vi "Main.vi"() -> ()   [LabVIEW 2019]
doc: "The myRIO Project template acquires acceleration data from the onboard accelerometer and displays the changes of acceleration values in a waveform chart."
uses:
  <vilib>/myRIO/Instrument Drivers/Onboard Devices/Accelerometer/typedefs/Accelerometer Reference.ctl
  <vilib>/myRIO/Common/Instrument Driver Framework/Utilities/typedefs/myRIO Generic Hardware Reference.ctl
  <vilib>/myRIO/Common/Instrument Driver Framework/Utilities/typedefs/Hardware Version Enum.ctl
  <vilib>/myRIO/Common/Instrument Driver Framework/Utilities/typedefs/myRIO v1.0 Reference.ctl
  <vilib>/myRIO/Common/Instrument Driver Framework/Utilities/typedefs/Generic FPGA Reference.ctl
  <vilib>/myRIO/Common/Instrument Driver Framework/myRIO v1.0/Accelerometer/typedefs/Accelerometer Channels List.ctl
  <vilib>/myRIO/Common/Instrument Driver Framework/myRIO v1.0/Accelerometer/typedefs/Accelerometer Channels Enum.ctl
  <vilib>/userDefined/High Color/nirio_resource_hc.ctl
  <vilib>/myRIO/Instrument Drivers/Onboard IO/AO/typedefs/AO Reference.ctl
  <vilib>/myRIO/Common/Instrument Driver Framework/myRIO v1.0/AO/typedefs/AO Channels List.ctl
  <vilib>/myRIO/Common/Instrument Driver Framework/myRIO v1.0/AO/typedefs/AO Channels Enum.ctl
  <vilib>/myRIO/Common/Instrument Driver Framework/Utilities/typedefs/Analog Scaling Constants List.ctl
  <vilib>/myRIO/Common/Instrument Driver Framework/Utilities/typedefs/Analog Scaling Constants.ctl
  <vilib>/myRIO/Common/Instrument Driver Framework/Utilities/vis/Is FPGA Ref Available.vi
  <vilib>/myRIO/Common/Instrument Driver Framework/myRIO v1.0/Accelerometer/vis/myRIO v1.1 Open Accelerometer.vi
  <vilib>/myRIO/Instrument Drivers/Onboard Devices/Accelerometer/vis/Read.vi
  <vilib>/myRIO/Common/Instrument Driver Framework/myRIO v1.0/AO/vis/myRIO v1.1 Open AO.vi
  <vilib>/myRIO/Instrument Drivers/Onboard IO/AO/vis/Write.vi
  <vilib>/myRIO/Common/Instrument Driver Framework/Utilities/vis/Validate Channels.vi
  <vilib>/myRIO/Common/Instrument Driver Framework/myRIO v1.0/Accelerometer/vis/myRIO v1.0 Reserve Accelerometer.vi
  <vilib>/myRIO/Common/Instrument Driver Framework/myRIO v1.0/UART/vis/myRIO v1.0 Close UART.vi
  <vilib>/myRIO/Common/Instrument Driver Framework/myRIO v1.0/AO/vis/myRIO v1.0 Reserve AO.vi
  <vilib>/myRIO/Common/Instrument Driver Framework/myRIO v1.0/Resource Manager/vis/myRIO v1.0 Reserve Channel List.vi
  <vilib>/myRIO/Common/Instrument Driver Framework/myRIO v1.0/Accelerometer/vis/myRIO v1.0 Build MUX Configuration Accelerometer.vi
  <vilib>/myRIO/Common/Instrument Driver Framework/myRIO v1.0/AO/vis/myRIO v1.0 Build MUX Configuration AO.vi
  <vilib>/myRIO/Common/Instrument Driver Framework/myRIO v1.0/Resource Manager/vis/myRIO v1.0 Reserve Channel.vi
  <vilib>/myRIO/Common/Instrument Driver Framework/myRIO v1.0/Resource Manager/vis/myRIO v1.0 Unreserve Channel.vi
  <vilib>/myRIO/Common/Instrument Driver Framework/myRIO v1.0/Resource Manager/vis/myRIO v1.0 Build Mutex Name.vi
  <vilib>/Utility/VariantDataType/GetNumericInfo.vi
  <vilib>/Utility/error.llb/Error Cluster From Error Code.vi
  <vilib>/myRIO/Common/Instrument Driver Framework/myRIO v1.0/myRIO v1.1 Open.vi
  <vilib>/myRIO/Common/Instrument Driver Framework/myRIO v1.0/AO/vis/myRIO v1.0 Get Scaling Constants AO.vi
  <vilib>/myRIO/Common/Instrument Driver Framework/Utilities/vis/IO Manager.vi
  <vilib>/myRIO/Common/Instrument Driver Framework/Utilities/vis/Configuration Manager.vi
  <vilib>/myRIO/Common/Instrument Driver Framework/myRIO v1.0/myRIO v1.0 Close.vi
  <vilib>/myRIO/Common/Instrument Driver Framework/myRIO v1.0/AO/vis/myRIO v1.0 Write AO.vi
  <vilib>/myRIO/Common/Instrument Driver Framework/myRIO v1.0/Accelerometer/vis/myRIO v1.0 Get Scaling Constant Accelerometer.vi
  <vilib>/myRIO/Common/Instrument Driver Framework/myRIO v1.0/Accelerometer/vis/myRIO v1.0 Read Accelerometer.vi
  <vilib>/myRIO/Common/Instrument Driver Framework/Utilities/vis/FPGA Ref Manager.vi
  <vilib>/myRIO/Common/Instrument Driver Framework/myRIO v1.0/myRIO v1.0 Reset FPGA.vi
  <vilib>/myRIO/Common/Instrument Driver Framework/myRIO v1.0/IRQ/vis/myRIO v1.0 IRQ Info FGV.vi
  <vilib>/myRIO/Common/Instrument Driver Framework/myRIO v1.0/IRQ/vis/myRIO v1.0 Timer IRQ Info FGV.vi
  <vilib>/myRIO/Common/Instrument Driver Framework/myRIO v1.0/IRQ/vis/myRIO v1.0 ISR Agent.vi
  <vilib>/myRIO/Instrument Drivers/Utilities/vis/Reset Index.vi
  <vilib>/myRIO/Common/Instrument Driver Framework/myRIO v1.0/Resource Manager/vis/myRIO v1.0 Block Write Resource Manager.vi
  <vilib>/myRIO/Express VI/Onboard IO/AO/AO Express VI.xnode
  <vilib>/myRIO/Instrument Drivers/Onboard IO/AO/vis/myRIO AO Open.xnode
  <vilib>/myRIO/Express VI/Onboard Devices/Accelerometer/Accelerometer Express VI.xnode
  <vilib>/myRIO/Instrument Drivers/Onboard Devices/Accelerometer/vis/myRIO Accelerometer Open.xnode
  <vilib>/myRIO/Instrument Drivers/Utilities/Utilities.lvlib
  <vilib>/myRIO/Instrument Drivers/Onboard Devices/Accelerometer/Accelerometer.lvlib
  <vilib>/myRIO/Instrument Drivers/Onboard IO/AO/AO.lvlib
panel:
  in  "Numeric 4":dbl
  in  "Numeric 3":dbl
  out "Array":i32[](array[numeric])
  in  "input array   4":dbl[](array[numeric])
  out "Numeric":i32
  out "Acceleration":T1(graph)
  out "error out":errorcluster
  in  "Stop":bool
  # "Overview: The myRIO Project template acquires acceleration data from the onboard accelerometer and displays the changes of acceleration values in a waveform chart.\nInstructions:\n1. Check the myRIO target IP address in the project and make sure the target IP address is correct. \n2. Run this VI."
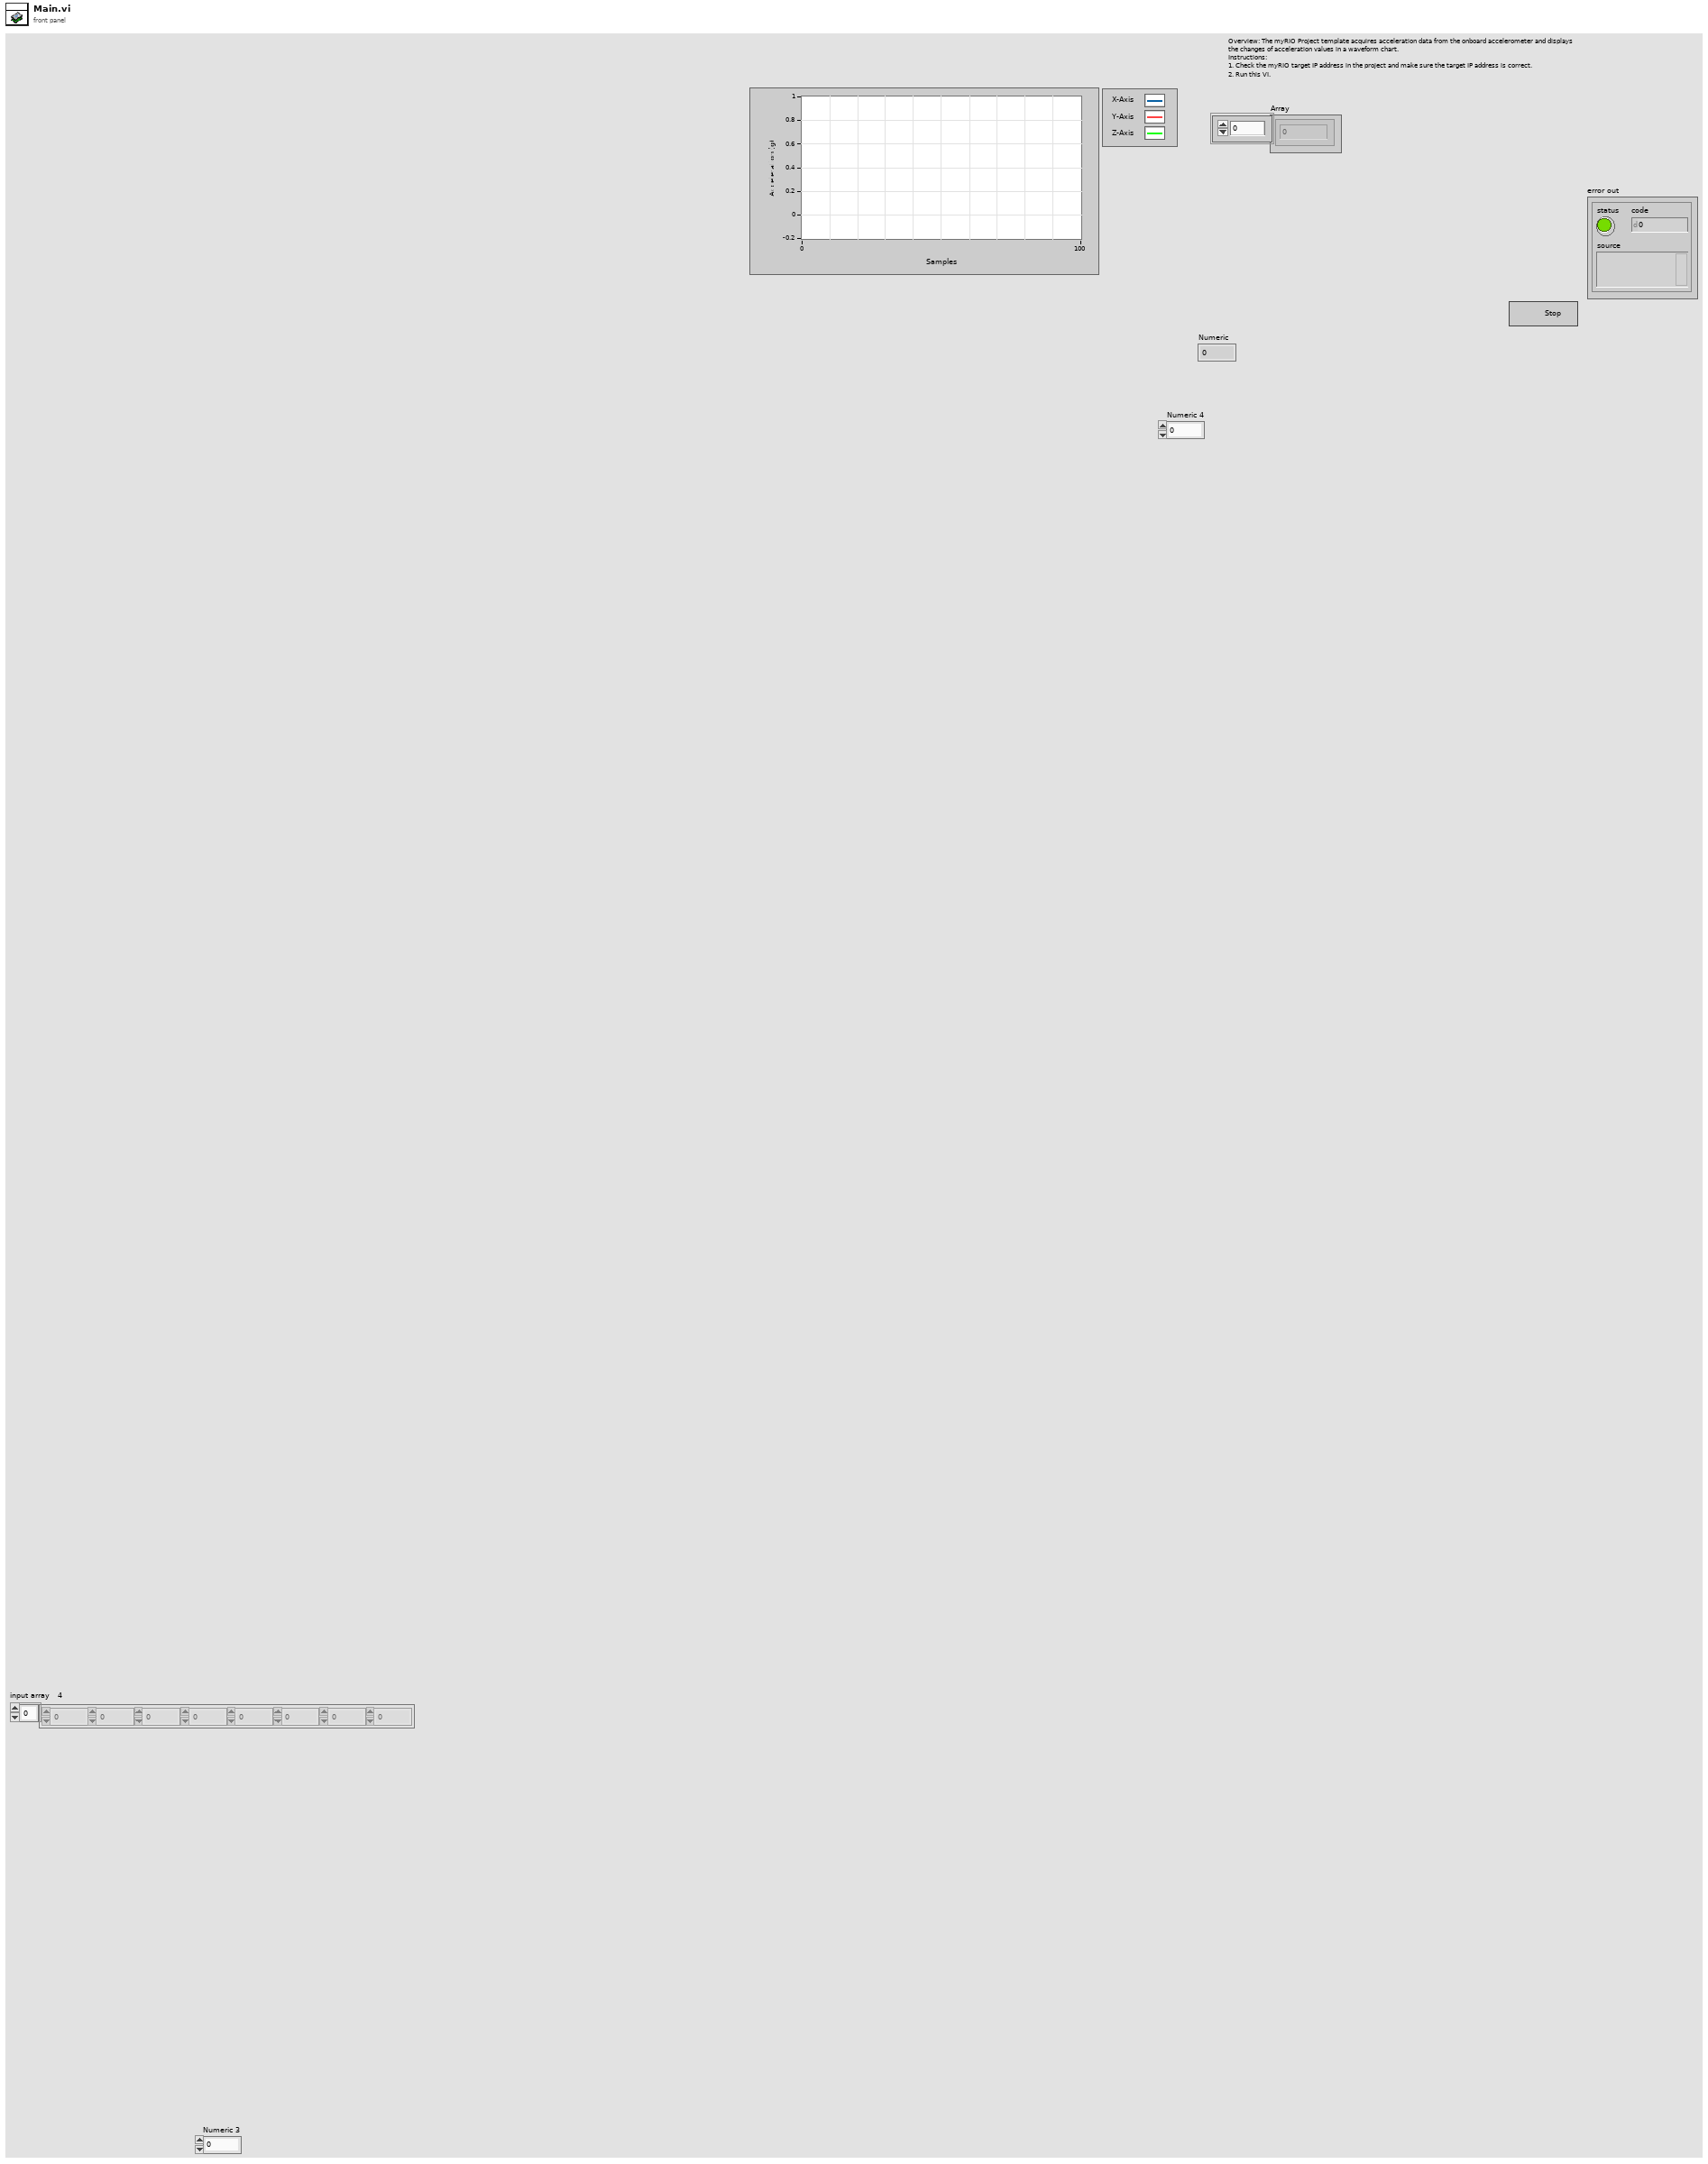
[diagram p1: front panel]
types:
  T1 = cluster{"X-Axis":dbl, "Y-Axis":dbl, "Z-Axis":dbl}
  T2 = typedef "Accelerometer.lvlib/Accelerometer Reference.ctl" = cluster{"myRIO Reference":T3, "Accelerometer Channels List":T7, "LSB Weight":dbl}
  T3 = typedef "myRIO Generic Hardware Reference.ctl" = cluster{"myRIO Model":T4, "myRIO Hardware Reference":T5}
  T4 = typedef "Hardware Version Enum.ctl" = enum16{"Unknown", "myRIO-1900", "myRIO-1950", "roboRIO", "NI ELVIS RIO CM", "ELVIS III"}
  T5 = typedef "myRIO v1.0 Reference.ctl" = cluster{"Generic FPGA Reference":T6, "Allow multiple opens":bool}
  T6 = typedef "Generic FPGA Reference.ctl" = refnum<k20>
  T7 = typedef "Accelerometer Channels List.ctl" = T8[]
  T8 = typedef "Accelerometer Channels Enum.ctl" = enum16{"Not Connected", "X-Axis", "Y-Axis", "Z-Axis"}
  T9 = typedef "nirio_resource_hc.ctl" = tag
  T10 = typedef "AO.lvlib/AO Reference.ctl" = cluster{"myRIO Reference":T3, "AO Channel List":T11, "AO Scaling Constant List":T13}
  T11 = typedef "AO Channels List.ctl" = T12[]
  T12 = typedef "AO Channels Enum.ctl" = enum16{"Not Connected", "AudioOut/Left", "AudioOut/Right", "C/AO0", "C/AO1", "A/AO0", "A/AO1", "B/AO0", "B/AO1"}
  T13 = typedef "Analog Scaling Constants List.ctl" = T14[]
  T14 = typedef "Analog Scaling Constants.ctl" = cluster{"LSB Weight (Volts)":dbl, "Offset (Volts)":dbl, "Signed?":bool}
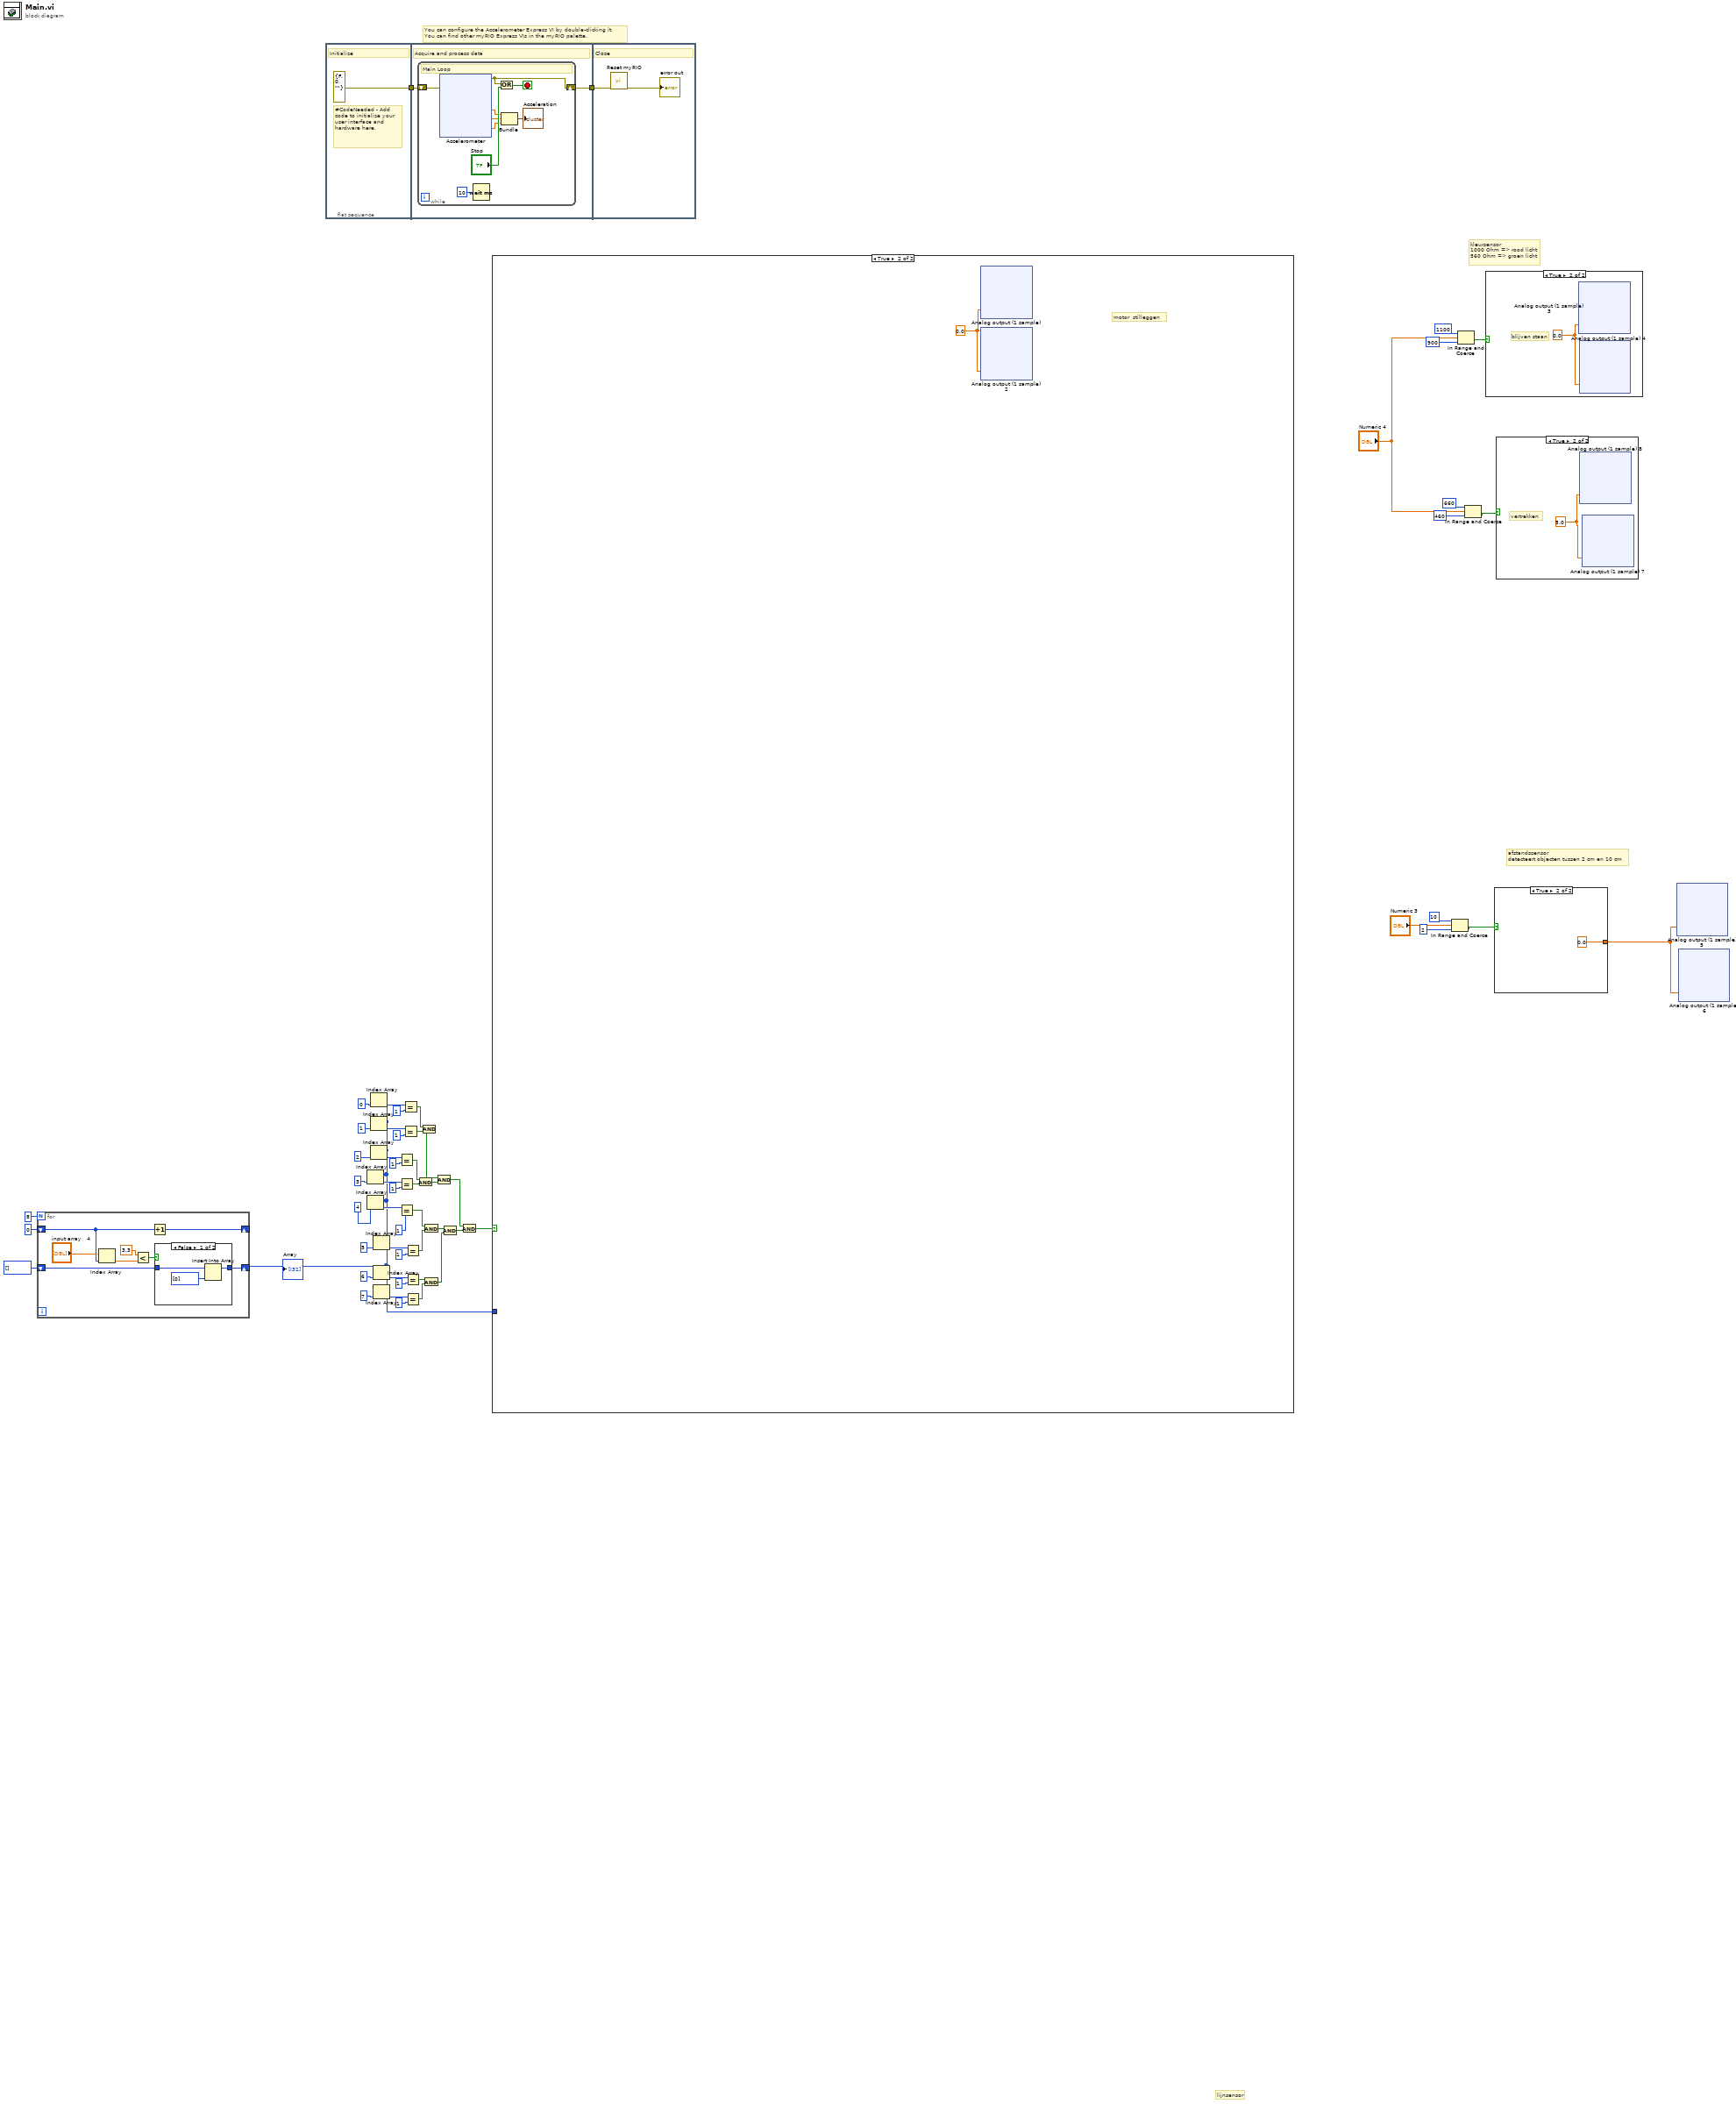
[diagram p0: block diagram]
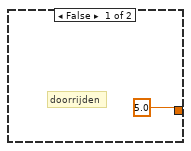
[diagram p4: hidden frame]
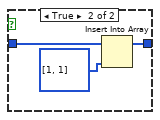
[diagram p5: hidden frame]
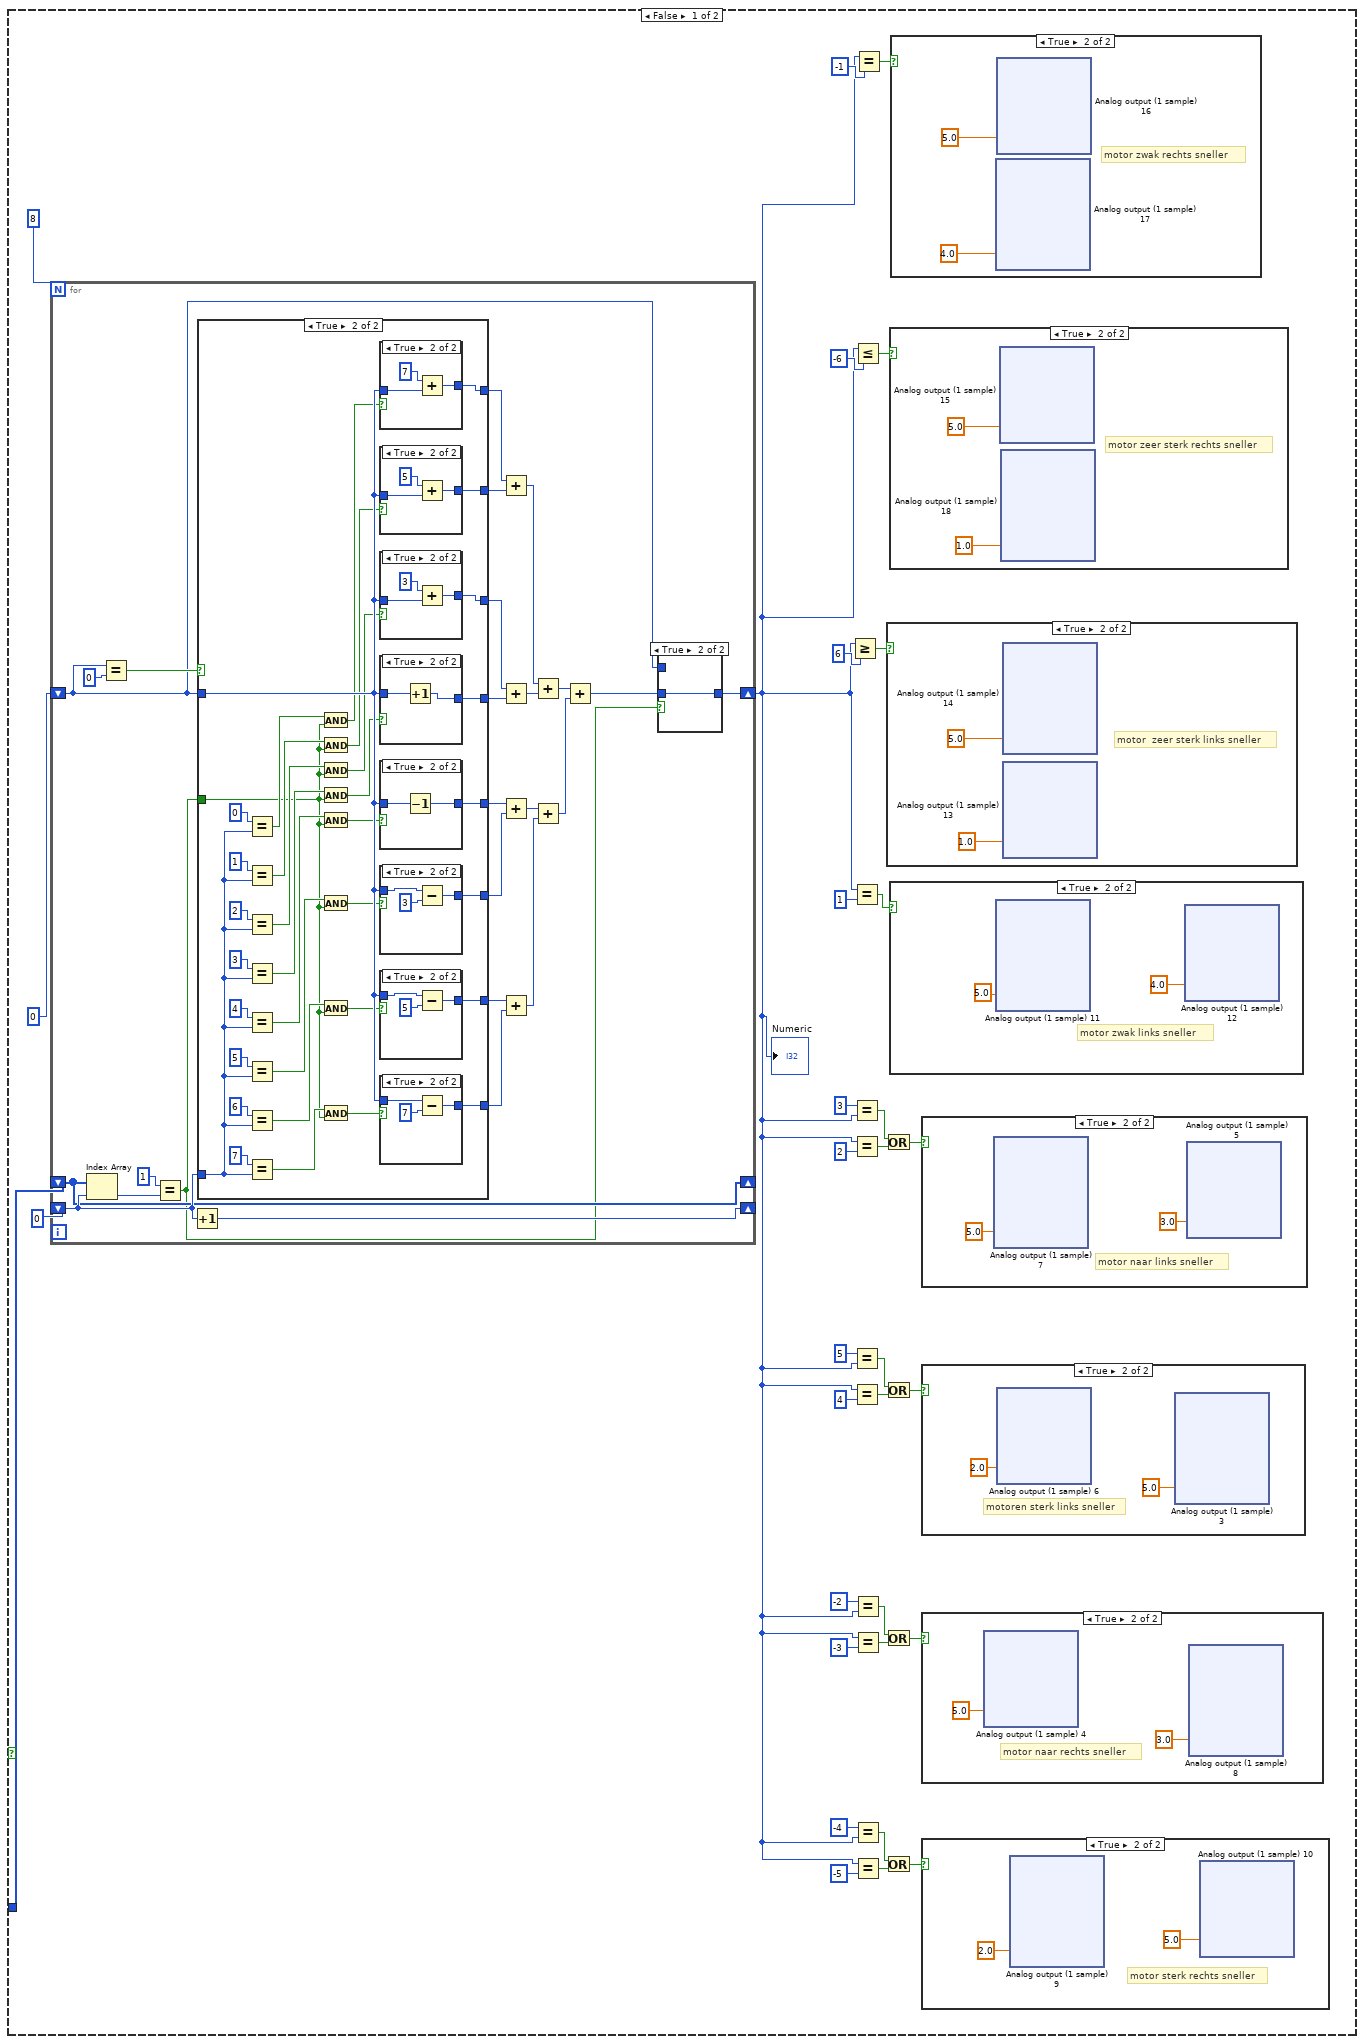
[diagram p6: hidden frame]
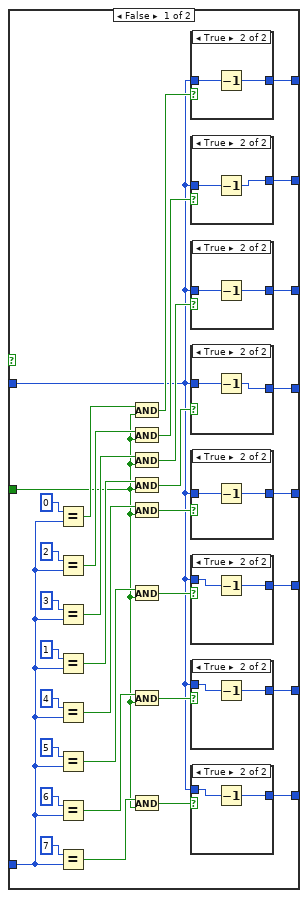
[diagram p16: hidden frame]
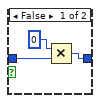
[diagram p17: hidden frame]
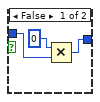
[diagram p18: hidden frame]
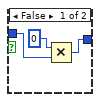
[diagram p19: hidden frame]
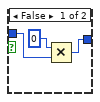
[diagram p20: hidden frame]
diagram:
  # "kleursensor    \n1000 Ohm => rood licht\n560 Ohm => groen licht"
  # "afstandssensor\ndetecteert objecten tussen 2 cm en 10 cm"
  # "lijnsensor"
  # "You can configure the Accelerometer Express VI by double-clicking it.\nYou can find other myRIO Express VIs in the myRIO palette."
  n1 = for {
    N: 8 -> [_]
    shift-right: [w64] -> w13
    shift-left: i32[] [] -> [w65]
    shift-right: [w61] -> _
    shift-left: 0 -> [w60]
    n2 = Index Array(array="input array   4", index=w60) -> (element=w58:dbl)
    n3 = Less?(x=3.3, y=w58) -> (x < y?=w63:bool)
    n4 = Increment(x=w60) -> (x+1=w61:i32)
    n5 = case shown="False" w63 {
      tunnel: w65 -> [w67 w69]
      tunnel: [w68 w71] -> w64
      frame False {
        n6 = Insert Into Array(array=w67, new element=i32[] [0]) -> (w68:i32[])  [unwired: 1 in]
      }
      frame True {
        n7 = Insert Into Array(array=w69, new element=i32[] [1, 1]) -> (w71:i32[])  [unwired: 1 in]
      }
    }
  }
  "Array" <- w13
  n8 = flat-sequence {
    tunnel: [errorcluster {"status"=FALSE, "code"=0, "source"=""} ("error in (no error)")] -> w57
    tunnel: w57 -> [w74]
    tunnel: [w73] -> w56
    tunnel: w56 -> [w124]
    frame #0 {
      # "#CodeNeeded - Add code to initialize your user interface and hardware here."
      # "Initialize"
    }
    frame #1 {
      # "Acquire and process data"
      n9 = while {
        shift-right: [w78] -> w73
        shift-left: w74 -> [w79]
        stop <- w82 stop-if-true
        # "Main Loop"
        n10 = xnode "Accelerometer"("error in (no error)"=w79) -> ("X-Axis"=w77:dbl, "Y-Axis"=w76:dbl, "Z-Axis"=w75:dbl, "error out"=w78:errorcluster)
        n11 = Wait (ms)(milliseconds to wait=u32 10) -> ()  [unwired: 1 out]
        n12 = Or(x=w78, y="Stop") -> (x .or. y?=w82:bool)
        n13 = Bundle("X-Axis"=w77, "Y-Axis"=w76, "Z-Axis"=w75) -> (→"Acceleration":T1)  [unwired: 1 in]
      }
    }
    frame #2 {
      # "Close"
      n14 = call <vilib>:"Reset myRIO.vi"("error in (no error)"=w124) -> ("error out"=→"error out":errorcluster)  [unwired: 10 in]
    }
  }
  n15 = Index Array(array=w13, index=3) -> (element=w52:i32)
  n16 = Index Array(array=w13, index=4) -> (element=w46:i32)
  n17 = Index Array(array=w13, index=0) -> (element=w34:i32)
  n18 = Index Array(array=w13, index=1) -> (element=w55:i32)
  n19 = Index Array(array=w13, index=2) -> (element=w49:i32)
  n20 = Index Array(array=w13, index=5) -> (element=w43:i32)
  n21 = Index Array(array=w13, index=6) -> (element=w40:i32)
  n22 = Index Array(array=w13, index=7) -> (element=w37:i32)
  n23 = Equal?(x=w49, y=1) -> (x = y?=w29:bool)
  n24 = Equal?(x=w52, y=1) -> (x = y?=w28:bool)
  n25 = Equal?(x=w46, y=1) -> (x = y?=w27:bool)
  n26 = Equal?(x=w34, y=1) -> (x = y?=w31:bool)
  n27 = Equal?(x=w55, y=1) -> (x = y?=w30:bool)
  n28 = Equal?(x=w43, y=1) -> (x = y?=w26:bool)
  n29 = Equal?(x=w40, y=1) -> (x = y?=w25:bool)
  n30 = Equal?(x=w37, y=1) -> (x = y?=w24:bool)
  n31 = And(x=w29, y=w28) -> (x .and. y?=w22:bool)
  n32 = And(x=w31, y=w30) -> (x .and. y?=w23:bool)
  n33 = And(x=w27, y=w26) -> (x .and. y?=w21:bool)
  n34 = And(x=w25, y=w24) -> (x .and. y?=w20:bool)
  n35 = And(x=w23, y=w22) -> (x .and. y?=w19:bool)
  n36 = And(x=w21, y=w20) -> (x .and. y?=w18:bool)
  n37 = And(x=w19, y=w18) -> (x .and. y?=w17:bool)
  n38 = case shown="True" w17 {
    tunnel: w13 -> [w126 _]
    frame False {
      n39 = for {
        N: 8 -> [_]
        shift-right: [w776] -> _
        shift-left: 0 -> [w790]
        shift-right: [w768] -> w125
        shift-left: 0 -> [w769]
        shift-right: [w781] -> _
        shift-left: w126 -> [w781]
        n40 = Index Array(array=w781, index=w790) -> (element=w780:i32)
        n41 = Equal?(x=w769, y=0) -> (x = y?=w777:bool)
        n42 = Equal?(x=1, y=w780) -> (x = y?=w767:bool)
        n43 = Increment(x=w790) -> (x+1=w776:i32)
        n44 = case shown="True" w777 {
          tunnel: w790 -> [w800 w886]
          tunnel: [w794 w885] -> w789
          tunnel: [w801 w884] -> w788
          tunnel: [w802 w883] -> w787
          tunnel: [w803 w882] -> w786
          tunnel: w769 -> [w793 w881]
          tunnel: w767 -> [w799 w872]
          tunnel: [w797 w871] -> w775
          tunnel: [w798 w870] -> w774
          tunnel: [w795 w869] -> w772
          tunnel: [w796 w868] -> w771
          frame False {
            n45 = Equal?(x=0, y=w800) -> (x = y?=w820:bool)
            n46 = Equal?(x=2, y=w800) -> (x = y?=w826:bool)
            n47 = Equal?(x=3, y=w800) -> (x = y?=w827:bool)
            n48 = Equal?(x=1, y=w800) -> (x = y?=w812:bool)
            n49 = Equal?(x=4, y=w800) -> (x = y?=w824:bool)
            n50 = Equal?(x=5, y=w800) -> (x = y?=w825:bool)
            n51 = Equal?(x=6, y=w800) -> (x = y?=w823:bool)
            n52 = Equal?(x=7, y=w800) -> (x = y?=w822:bool)
            n53 = And(x=w820, y=w799) -> (x .and. y?=w804:bool)
            n54 = And(x=w826, y=w799) -> (x .and. y?=w806:bool)
            n55 = And(x=w827, y=w799) -> (x .and. y?=w807:bool)
            n56 = And(x=w812, y=w799) -> (x .and. y?=w805:bool)
            n57 = And(x=w824, y=w799) -> (x .and. y?=w808:bool)
            n58 = And(x=w825, y=w799) -> (x .and. y?=w809:bool)
            n59 = And(x=w823, y=w799) -> (x .and. y?=w810:bool)
            n60 = And(x=w822, y=w799) -> (x .and. y?=w811:bool)
            n61 = case shown="True" w804 {
              tunnel: [w829 w832] -> w798
              tunnel: w793 -> [w828 w831]
              frame False {
                n62 = Multiply(x=0, y=w828) -> (x*y=w829:i32)
              }
              frame True {
                n63 = Decrement(x=w831) -> (x-1=w832:i32)
              }
            }
            n64 = case shown="True" w806 {
              tunnel: [w860 w861] -> w797
              tunnel: w793 -> [w859 w862]
              frame False {
                n65 = Multiply(x=0, y=w859) -> (x*y=w860:i32)
              }
              frame True {
                n66 = Decrement(x=w862) -> (x-1=w861:i32)
              }
            }
            n67 = case shown="True" w807 {
              tunnel: [w854 w857] -> w796
              tunnel: w793 -> [w853 w856]
              frame False {
                n68 = Multiply(x=0, y=w853) -> (x*y=w854:i32)
              }
              frame True {
                n69 = Decrement(x=w856) -> (x-1=w857:i32)
              }
            }
            n70 = case shown="True" w805 {
              tunnel: [w864 w867] -> w795
              tunnel: w793 -> [w863 w866]
              frame False {
                n71 = Multiply(x=0, y=w863) -> (x*y=w864:i32)
              }
              frame True {
                n72 = Decrement(x=w866) -> (x-1=w867:i32)
              }
            }
            n73 = case shown="True" w808 {
              tunnel: [w849 w852] -> w794
              tunnel: w793 -> [w848 w851]
              frame False {
                n74 = Multiply(x=0, y=w848) -> (x*y=w849:i32)
              }
              frame True {
                n75 = Decrement(x=w851) -> (x-1=w852:i32)
              }
            }
            n76 = case shown="True" w809 {
              tunnel: [w839 w842] -> w801
              tunnel: w793 -> [w838 w841]
              frame False {
                n77 = Multiply(x=0, y=w838) -> (x*y=w839:i32)
              }
              frame True {
                n78 = Decrement(x=w841) -> (x-1=w842:i32)
              }
            }
            n79 = case shown="True" w810 {
              tunnel: [w844 w847] -> w802
              tunnel: w793 -> [w843 w846]
              frame False {
                n80 = Multiply(x=0, y=w843) -> (x*y=w844:i32)
              }
              frame True {
                n81 = Decrement(x=w846) -> (x-1=w847:i32)
              }
            }
            n82 = case shown="True" w811 {
              tunnel: [w833 w837] -> w803
              tunnel: w793 -> [w834 w836]
              frame False {
                n83 = Multiply(x=0, y=w834) -> (x*y=w833:i32)
              }
              frame True {
                n84 = Decrement(x=w836) -> (x-1=w837:i32)
              }
            }
          }
          frame True {
            n85 = Equal?(x=0, y=w886) -> (x = y?=w895:bool)
            n86 = Equal?(x=1, y=w886) -> (x = y?=w887:bool)
            n87 = Equal?(x=2, y=w886) -> (x = y?=w901:bool)
            n88 = Equal?(x=3, y=w886) -> (x = y?=w902:bool)
            n89 = Equal?(x=4, y=w886) -> (x = y?=w899:bool)
            n90 = Equal?(x=5, y=w886) -> (x = y?=w900:bool)
            n91 = Equal?(x=6, y=w886) -> (x = y?=w898:bool)
            n92 = Equal?(x=7, y=w886) -> (x = y?=w897:bool)
            n93 = And(x=w895, y=w872) -> (x .and. y?=w873:bool)
            n94 = And(x=w887, y=w872) -> (x .and. y?=w874:bool)
            n95 = And(x=w901, y=w872) -> (x .and. y?=w875:bool)
            n96 = And(x=w902, y=w872) -> (x .and. y?=w876:bool)
            n97 = And(x=w899, y=w872) -> (x .and. y?=w877:bool)
            n98 = And(x=w900, y=w872) -> (x .and. y?=w878:bool)
            n99 = And(x=w898, y=w872) -> (x .and. y?=w879:bool)
            n100 = And(x=w897, y=w872) -> (x .and. y?=w880:bool)
            n101 = case shown="True" w873 {
              tunnel: w881 -> [w903 w907]
              tunnel: [w904 w906] -> w870
              frame False {
                n102 = Multiply(x=0, y=w903) -> (x*y=w904:i32)
              }
              frame True {
                n103 = Add(x=7, y=w907) -> (x+y=w906:i32)
              }
            }
            n104 = case shown="True" w874 {
              tunnel: w881 -> [w943 w946]
              tunnel: [w944 w947] -> w871
              frame False {
                n105 = Multiply(x=0, y=w943) -> (x*y=w944:i32)
              }
              frame True {
                n106 = Add(x=5, y=w946) -> (x+y=w947:i32)
              }
            }
            n107 = case shown="True" w875 {
              tunnel: w881 -> [w937 w941]
              tunnel: [w938 w940] -> w868
              frame False {
                n108 = Multiply(x=0, y=w937) -> (x*y=w938:i32)
              }
              frame True {
                n109 = Add(x=3, y=w941) -> (x+y=w940:i32)
              }
            }
            n110 = case shown="True" w876 {
              tunnel: w881 -> [w933 w936]
              tunnel: [w932 w935] -> w869
              frame False {
                n111 = Multiply(x=0, y=w933) -> (x*y=w932:i32)
              }
              frame True {
                n112 = Increment(x=w936) -> (x+1=w935:i32)
              }
            }
            n113 = case shown="True" w877 {
              tunnel: w881 -> [w927 w931]
              tunnel: [w928 w930] -> w885
              frame False {
                n114 = Multiply(x=0, y=w927) -> (x*y=w928:i32)
              }
              frame True {
                n115 = Decrement(x=w931) -> (x-1=w930:i32)
              }
            }
            n116 = case shown="True" w878 {
              tunnel: w881 -> [w916 w918]
              tunnel: [w915 w920] -> w884
              frame False {
                n117 = Multiply(x=0, y=w916) -> (x*y=w915:i32)
              }
              frame True {
                n118 = Subtract(x=w918, y=3) -> (x-y=w920:i32)
              }
            }
            n119 = case shown="True" w879 {
              tunnel: w881 -> [w922 w924]
              tunnel: [w921 w925] -> w883
              frame False {
                n120 = Multiply(x=0, y=w922) -> (x*y=w921:i32)
              }
              frame True {
                n121 = Subtract(x=w924, y=5) -> (x-y=w925:i32)
              }
            }
            n122 = case shown="True" w880 {
              tunnel: w881 -> [w909 w912]
              tunnel: [w910 w913] -> w882
              frame False {
                n123 = Multiply(x=0, y=w909) -> (x*y=w910:i32)
              }
              frame True {
                n124 = Subtract(x=w912, y=7) -> (x-y=w913:i32)
              }
            }
          }
        }
        n125 = Add(x=w774, y=w775) -> (x+y=w773:i32)
        n126 = Add(x=w771, y=w772) -> (x+y=w770:i32)
        n127 = Add(x=w789, y=w788) -> (x+y=w784:i32)
        n128 = Add(x=w787, y=w786) -> (x+y=w785:i32)
        n129 = Add(x=w773, y=w770) -> (x+y=w783:i32)
        n130 = Add(x=w784, y=w785) -> (x+y=w782:i32)
        n131 = Add(x=w783, y=w782) -> (x+y=w766:i32)
        n132 = case shown="True" w767 {
          tunnel: w769 -> [w791 _]
          tunnel: [w791 w792] -> w768
          tunnel: w766 -> [_ w792]
          frame False {
          }
          frame True {
          }
        }
      }
      "Numeric" <- w125
      n133 = Greater Or Equal?(x=w125, y=6) -> (x >= y?=w152:bool)
      n134 = Equal?(x=w125, y=1) -> (x = y?=w153:bool)
      n135 = Equal?(x=3, y=w125) -> (x = y?=w143:bool)
      n136 = Equal?(x=w125, y=2) -> (x = y?=w144:bool)
      n137 = Equal?(x=5, y=w125) -> (x = y?=w147:bool)
      n138 = Equal?(x=w125, y=4) -> (x = y?=w148:bool)
      n139 = Less Or Equal?(x=w125, y=-6) -> (x <= y?=w129:bool)
      n140 = Equal?(x=-2, y=w125) -> (x = y?=w137:bool)
      n141 = Equal?(x=w125, y=-3) -> (x = y?=w138:bool)
      n142 = Equal?(x=-4, y=w125) -> (x = y?=w133:bool)
      n143 = Equal?(x=w125, y=-5) -> (x = y?=w134:bool)
      n144 = Equal?(x=w125, y=-1) -> (x = y?=w131:bool)
      n145 = Or(x=w143, y=w144) -> (x .or. y?=w141:bool)
      n146 = Or(x=w147, y=w148) -> (x .or. y?=w149:bool)
      n147 = Or(x=w137, y=w138) -> (x .or. y?=w130:bool)
      n148 = Or(x=w133, y=w134) -> (x .or. y?=w127:bool)
      n149 = case shown="True" w152 {
        frame False {
        }
        frame True {
          # "motor  zeer sterk links sneller"
          n150 = xnode "Analog output (1 sample) 14"("A/AO0 (Pin 2)"=5.0) -> ()  [unwired: 1 in, 1 out]
          n151 = xnode "Analog output (1 sample) 13"("A/AO0 (Pin 2)"=1.0) -> ()  [unwired: 1 in, 1 out]
        }
      }
      n152 = case shown="True" w129 {
        frame False {
        }
        frame True {
          # "motor zeer sterk rechts sneller"
          n153 = xnode "Analog output (1 sample) 15"("A/AO0 (Pin 2)"=5.0) -> ()  [unwired: 1 in, 1 out]
          n154 = xnode "Analog output (1 sample) 18"("A/AO0 (Pin 2)"=1.0) -> ()  [unwired: 1 in, 1 out]
        }
      }
      n155 = case shown="True" w153 {
        frame False {
        }
        frame True {
          # "motor zwak links sneller"
          n156 = xnode "Analog output (1 sample) 11"("A/AO0 (Pin 2)"=5.0) -> ()  [unwired: 1 in, 1 out]
          n157 = xnode "Analog output (1 sample) 12"("A/AO0 (Pin 2)"=4.0) -> ()  [unwired: 1 in, 1 out]
        }
      }
      n158 = case shown="True" w131 {
        frame False {
        }
        frame True {
          # "motor zwak rechts sneller"
          n159 = xnode "Analog output (1 sample) 17"("A/AO0 (Pin 2)"=4.0) -> ()  [unwired: 1 in, 1 out]
          n160 = xnode "Analog output (1 sample) 16"("A/AO0 (Pin 2)"=5.0) -> ()  [unwired: 1 in, 1 out]
        }
      }
      n161 = case shown="True" w141 {
        frame False {
        }
        frame True {
          # "motor naar links sneller"
          n162 = xnode "Analog output (1 sample) 7"("A/AO0 (Pin 2)"=5.0) -> ()  [unwired: 1 in, 1 out]
          n163 = xnode "Analog output (1 sample) 5"("A/AO0 (Pin 2)"=3.0) -> ()  [unwired: 1 in, 1 out]
        }
      }
      n164 = case shown="True" w149 {
        frame False {
        }
        frame True {
          # "motoren sterk links sneller"
          n165 = xnode "Analog output (1 sample) 6"("A/AO0 (Pin 2)"=2.0) -> ()  [unwired: 1 in, 1 out]
          n166 = xnode "Analog output (1 sample) 3"("A/AO0 (Pin 2)"=5.0) -> ()  [unwired: 1 in, 1 out]
        }
      }
      n167 = case shown="True" w130 {
        frame False {
        }
        frame True {
          # "motor naar rechts sneller"
          n168 = xnode "Analog output (1 sample) 4"("A/AO0 (Pin 2)"=5.0) -> ()  [unwired: 1 in, 1 out]
          n169 = xnode "Analog output (1 sample) 8"("A/AO0 (Pin 2)"=3.0) -> ()  [unwired: 1 in, 1 out]
        }
      }
      n170 = case shown="True" w127 {
        frame False {
        }
        frame True {
          # "motor sterk rechts sneller"
          n171 = xnode "Analog output (1 sample) 9"("A/AO0 (Pin 2)"=2.0) -> ()  [unwired: 1 in, 1 out]
          n172 = xnode "Analog output (1 sample) 10"("A/AO0 (Pin 2)"=5.0) -> ()  [unwired: 1 in, 1 out]
        }
      }
    }
    frame True {
      w949 = 0.0
      # "motor  stilleggen"
      n173 = xnode "Analog output (1 sample)"("A/AO0 (Pin 2)"=w949) -> ()  [unwired: 1 in, 1 out]
      n174 = xnode "Analog output (1 sample) 2"("A/AO0 (Pin 2)"=w949) -> ()  [unwired: 1 in, 1 out]
    }
  }
  n175 = In Range and Coerce(upper limit=10, x="Numeric 3", lower limit=2) -> (In Range?=w9:bool)  [unwired: 1 out]
  n176 = In Range and Coerce(upper limit=1100, x="Numeric 4", lower limit=900) -> (In Range?=w5:bool)  [unwired: 1 out]
  n177 = In Range and Coerce(upper limit=660, x="Numeric 4", lower limit=460) -> (In Range?=w2:bool)  [unwired: 1 out]
  n178 = case shown="True" w5 {
    frame False {
    }
    frame True {
      w1024 = 0.0
      # "blijven staan"
      n179 = xnode "Analog output (1 sample) 3"("A/AO0 (Pin 2)"=w1024) -> ()  [unwired: 1 in, 1 out]
      n180 = xnode "Analog output (1 sample) 4"("A/AO0 (Pin 2)"=w1024) -> ()  [unwired: 1 in, 1 out]
    }
  }
  n181 = case shown="True" w9 {
    tunnel: [5.0 0.0] -> w12
    frame False {
      # "doorrijden"
    }
    frame True {
    }
  }
  n182 = case shown="True" w2 {
    frame False {
    }
    frame True {
      w1101 = 5.0
      # "vertrekken"
      n183 = xnode "Analog output (1 sample) 8"("A/AO0 (Pin 2)"=w1101) -> ()  [unwired: 1 in, 1 out]
      n184 = xnode "Analog output (1 sample) 7"("A/AO0 (Pin 2)"=w1101) -> ()  [unwired: 1 in, 1 out]
    }
  }
  n185 = xnode "Analog output (1 sample) 5"("A/AO0 (Pin 2)"=w12) -> ()  [unwired: 1 in, 1 out]
  n186 = xnode "Analog output (1 sample) 6"("A/AO0 (Pin 2)"=w12) -> ()  [unwired: 1 in, 1 out]
